vi "HardwareStart.vi"(8 "Error In":errorcluster, 10 "Hardware Configuration":T1={"DUT"={"Count"=1, "Wirings"=[], "Names"=[]}, "Log"={"Start"={"Trigger Type"=enum."Immediate", "Timer (sec)"=0.0, "Digital IO Line"=0, "Digital IO Edge"=enum."Rising"}, "Rollover"={"Trigger Type"=enum."None", "Timer (sec)"=0.0, "File Size (MB)"=0, "Digital IO Line"=0, "Digital IO Edge"=enum."Rising"}, "Stop"={"Trigger Type"=enum."None", "Timer (sec)"=0.0, "File Size (MB)"=0, "Digital IO Line"=0, "Digital IO Edge"=enum."Rising"}}, "Trigger"={"Input"={"Type"=enum."None", "Timeout (ms)"=0, "Delay (ms)"=0, "Digital IO Line (1-14)"=0, "Digital IO Mode"=enum."Falling"}, "Output"={"Type"=enum."None", "Delay (ms)"=0, "Digital IO Line (1-14)"=0, "Digital IO Mode"=enum."Falling", "Digital IO Pulse Width (sec)"=0.0}}, "Sources"=[], "Measures"=[]} {"Measures"."Count" min=1 step=1; "Trigger"."Output"."Digital IO Line (1-14)" min=1 max=14 step=1}, 11 "Keithley 2602 In":refnum<visa-resource-name>) -> (0 "Error Out":errorcluster, 3 "Keithley 2602 Out":refnum<visa-resource-name>)   [LabVIEW 2012]
uses:
  Setup.ctl
  DUTConfiguration.ctl
  driver/Public/Controls/SMUSense.ctl
  LogConfiguration.ctl
  LogStartConfiguration.ctl
  LogStartTriggerType.ctl
  LogDigitalIOTriggerEdge.ctl
  LogRolloverConfiguration.ctl
  LogRolloverTriggerType.ctl
  LogStopConfiguration.ctl
  LogStopTriggerType.ctl
  TriggerConfiguration.ctl
  TriggerInputConfiguration.ctl
  TriggerInputType.ctl
  driver/Public/Controls/TriggerMode.ctl
  TriggerOutputConfiguration.ctl
  TriggerOutputType.ctl
  SourceConfiguration.ctl
  SourceFunction.ctl
  MeasureConfiguration.ctl
  driver/Public/Controls/SMU.ctl
  HardwareAbortGlobalAction.ctl
  driver/Keithley-2602.lvlib
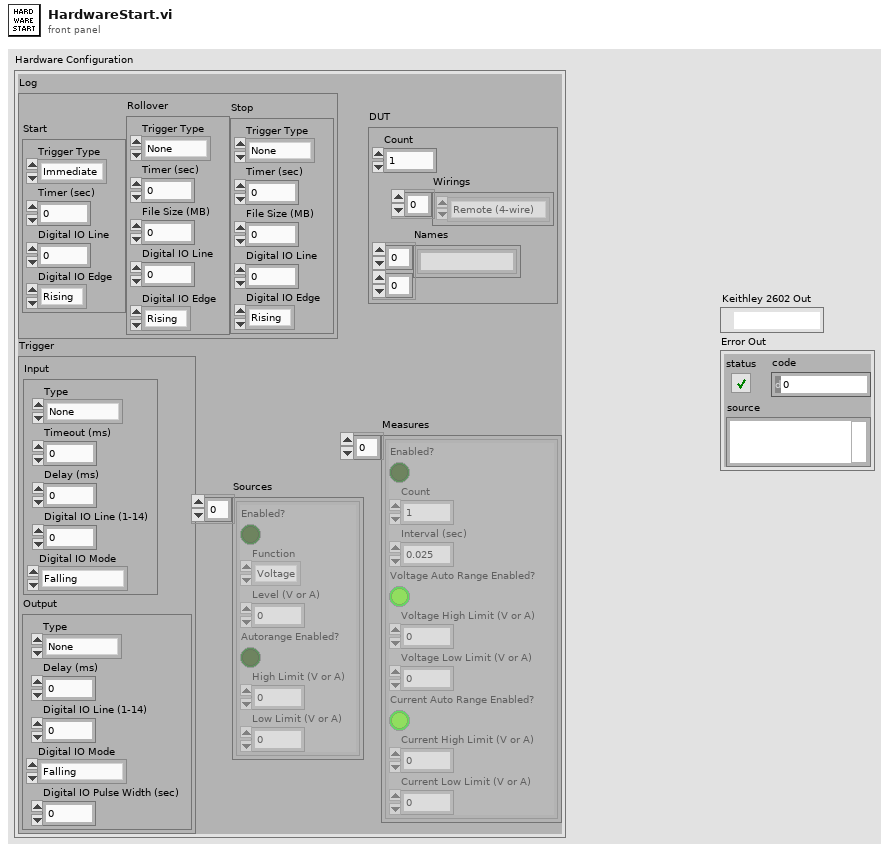
[diagram p1: front panel]
types:
  T1 = typedef "Setup.ctl" = cluster{"DUT":T2, "Log":T4, "Trigger":T12, "Sources":T18[], "Measures":T20[]}
  T2 = typedef "DUTConfiguration.ctl" = cluster{"Count":u32, "Wirings":T3[], "Names":string[][]}
  T3 = typedef "Keithley-2602.lvlib/SMUSense.ctl" = enum16{"Local (2-wire)", "Remote (4-wire)", "Calibration"}
  T4 = typedef "LogConfiguration.ctl" = cluster{"Start":T5, "Rollover":T8, "Stop":T10}
  T5 = typedef "LogStartConfiguration.ctl" = cluster{"Trigger Type":T6, "Timer (sec)":dbl, "Digital IO Line":u8, "Digital IO Edge":T7}
  T6 = typedef "LogStartTriggerType.ctl" = enum16{"Immediate", "User", "Timer", "Digital IO"}
  T7 = typedef "LogDigitalIOTriggerEdge.ctl" = enum16{"Rising", "Falling"}
  T8 = typedef "LogRolloverConfiguration.ctl" = cluster{"Trigger Type":T9, "Timer (sec)":dbl, "File Size (MB)":u32, "Digital IO Line":u8, "Digital IO Edge":T7}
  T9 = typedef "LogRolloverTriggerType.ctl" = enum16{"None", "Timer", "File Size", "Digital IO"}
  T10 = typedef "LogStopConfiguration.ctl" = cluster{"Trigger Type":T11, "Timer (sec)":dbl, "File Size (MB)":u32, "Digital IO Line":u8, "Digital IO Edge":T7}
  T11 = typedef "LogStopTriggerType.ctl" = enum16{"None", "User", "Timer", "File Size", "Digital IO"}
  T12 = typedef "TriggerConfiguration.ctl" = cluster{"Input":T13, "Output":T16}
  T13 = typedef "TriggerInputConfiguration.ctl" = cluster{"Type":T14, "Timeout (ms)":u32, "Delay (ms)":u32, "Digital IO Line (1-14)":u8, "Digital IO Mode":T15}
  T14 = typedef "TriggerInputType.ctl" = enum16{"None", "Digital IO", "Bus"}
  T15 = typedef "Keithley-2602.lvlib/TriggerMode.ctl" = enum16{"Falling", "Rising", "Either", "Synchronous"}
  T16 = typedef "TriggerOutputConfiguration.ctl" = cluster{"Type":T17, "Delay (ms)":u32, "Digital IO Line (1-14)":u8, "Digital IO Mode":T15, "Digital IO Pulse Width (sec)":dbl}
  T17 = typedef "TriggerOutputType.ctl" = enum16{"None", "Digital IO", "Bus"}
  T18 = typedef "SourceConfiguration.ctl" = cluster{"Enabled?":bool, "Function":T19, "Level (V or A)":dbl, "Autorange Enabled?":bool, "High Limit (V or A)":dbl, "Low Limit (V or A)":dbl}
  T19 = typedef "SourceFunction.ctl" = enum16{"Voltage", "Current"}
  T20 = typedef "MeasureConfiguration.ctl" = cluster{"Enabled?":bool, "Count":u8, "Interval (sec)":dbl, "Voltage Auto Range Enabled?":bool, "Voltage High Limit (V or A)":dbl, "Voltage Low Limit (V or A)":dbl, "Current Auto Range Enabled?":bool, "Current High Limit (V or A)":dbl, "Current Low Limit (V or A)":dbl}
  T21 = typedef "HardwareAbortGlobalAction.ctl" = enum16{"Set", "Get"}
  T22 = typedef "Keithley-2602.lvlib/SMU.ctl" = enum16{"A", "B"}
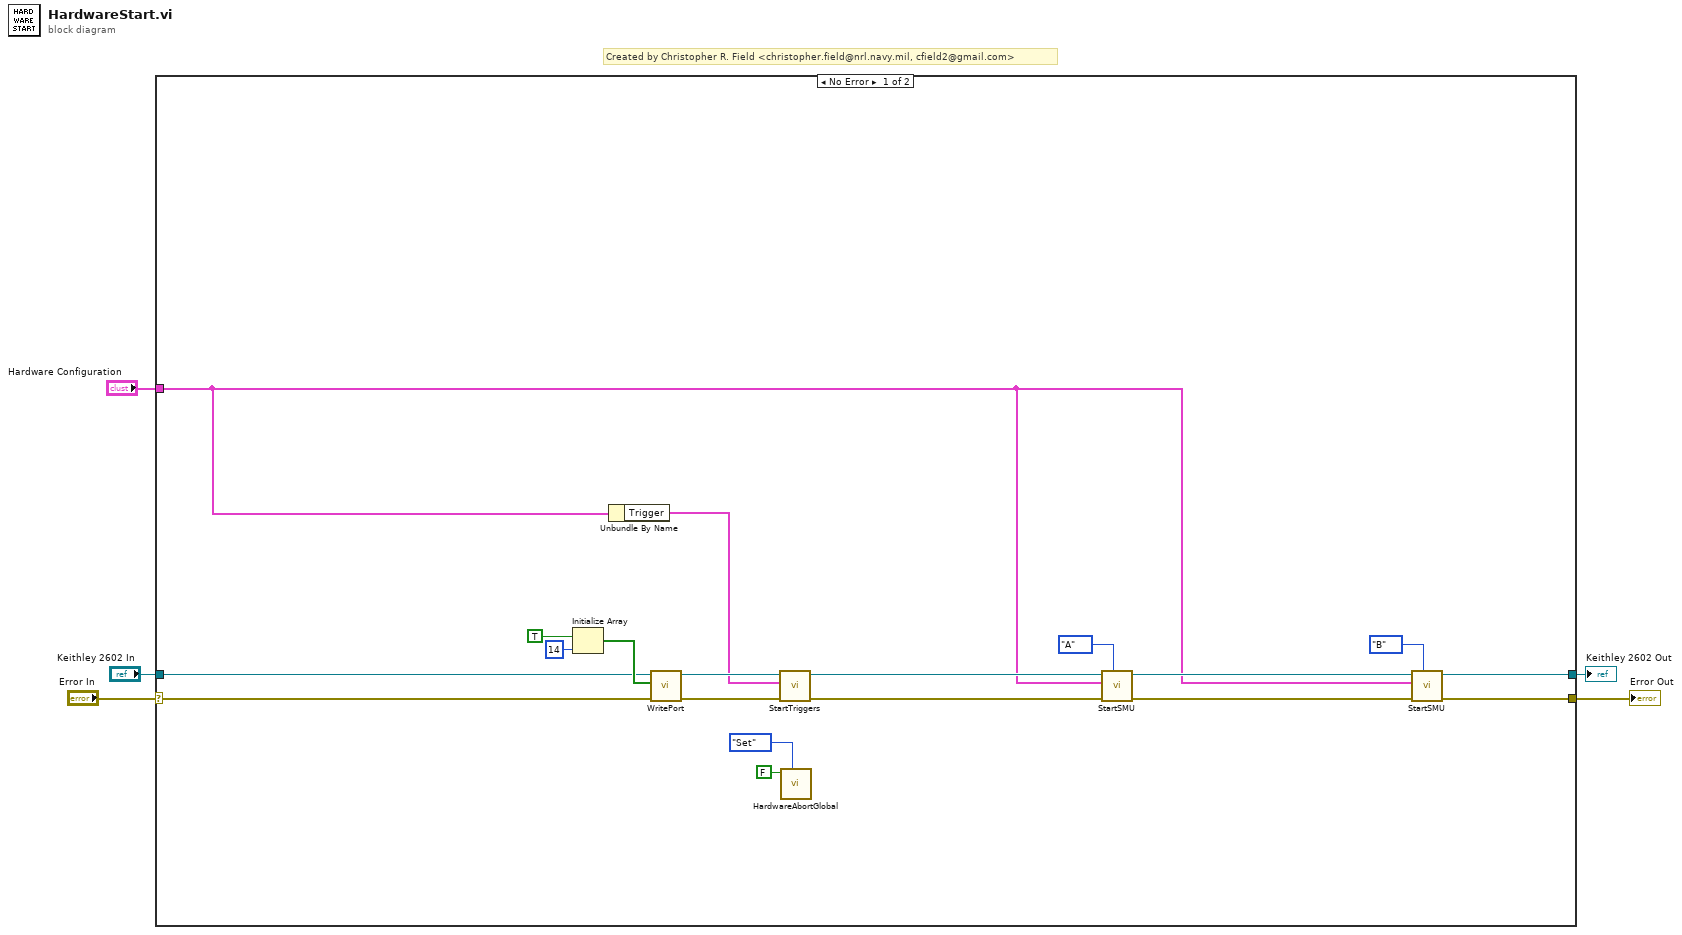
[diagram p0: block diagram]
diagram:
  # "Created by Christopher R. Field <christopher.field@nrl.navy.mil, cfield2@gmail.com>"
  n1 = case shown="No Error" "Error In" {
    selector: "Error In" -> [w12 w25]
    tunnel: "Keithley 2602 In" -> [w15 w26]
    tunnel: [w22 w26] -> w3
    tunnel: [w21 w25] -> w2
    tunnel: "Hardware Configuration" -> [w8 _]
    frame No Error {
      n2 = Initialize Array(TRUE, 14 ("dimension size")) -> (w16:bool[])
      n3 = Unbundle By Name(w8) -> ("Trigger"=w9:T12)
      n4 = call "WritePort.vi"("Error In"=w12, "Port"=w16, "Keithley 2602 In"=w15) -> ("Error Out"=w13:errorcluster, "Keithley 2602 Out"=w14:refnum<visa-resource-name>)  [unwired: 7 in]
      n5 = call "StartTriggers.vi"("Error In"=w13, "Trigger Configuration"=w9, "Keithley 2602 In"=w14) -> ("Error Out"=w19:errorcluster, "Keithley 2602 Out"=w20:refnum<visa-resource-name>)  [unwired: 7 in]
      n6 = call "HardwareAbortGlobal.vi"("Action"=HardwareAbortGlobalAction."Set", "Set Value"=FALSE) -> ()  [unwired: 9 in, 1 out]
      n7 = call "StartSMU.vi"("SMU"=SMU."A", "Error In"=w19, "Hardware Configuration"=w8, "Keithley 2602 In"=w20) -> ("Error Out"=w23:errorcluster, "Keithley 2602 Out"=w24:refnum<visa-resource-name>)  [unwired: 6 in]
      n8 = call "StartSMU.vi"("SMU"=SMU."B", "Error In"=w23, "Hardware Configuration"=w8, "Keithley 2602 In"=w24) -> ("Error Out"=w21:errorcluster, "Keithley 2602 Out"=w22:refnum<visa-resource-name>)  [unwired: 6 in]
    }
    frame Error {
    }
  }
  "Keithley 2602 Out" <- w3
  "Error Out" <- w2
